vi "_PC_Daemon_Laser_Set_Status.vi"(5 "eng_mode_str":refnum<vi>, 7 "function":enum16{"none", "init", "set", "get"}(ring), 8 "error in (no error)":errorcluster, 10 "LaserSetting in":T1={"Energy"=50.0, "Freq"=100.0, "Emission"=FALSE, "TriggerSource"=enum."Internal", "Time Stamp"=timestamp(0 s since 1904-01-01)}, 11 "refnum cluster in":T2) -> (0 "error out":errorcluster, 2 "LaserSetting out":T1={"Energy"=50.0, "Freq"=100.0, "Emission"=FALSE, "TriggerSource"=enum."Internal", "Time Stamp"=timestamp(0 s since 1904-01-01)})   [LabVIEW 2018]
uses:
  RT/ControlLoop/Laser/Ctl/_ctl_LaserParam.ctl
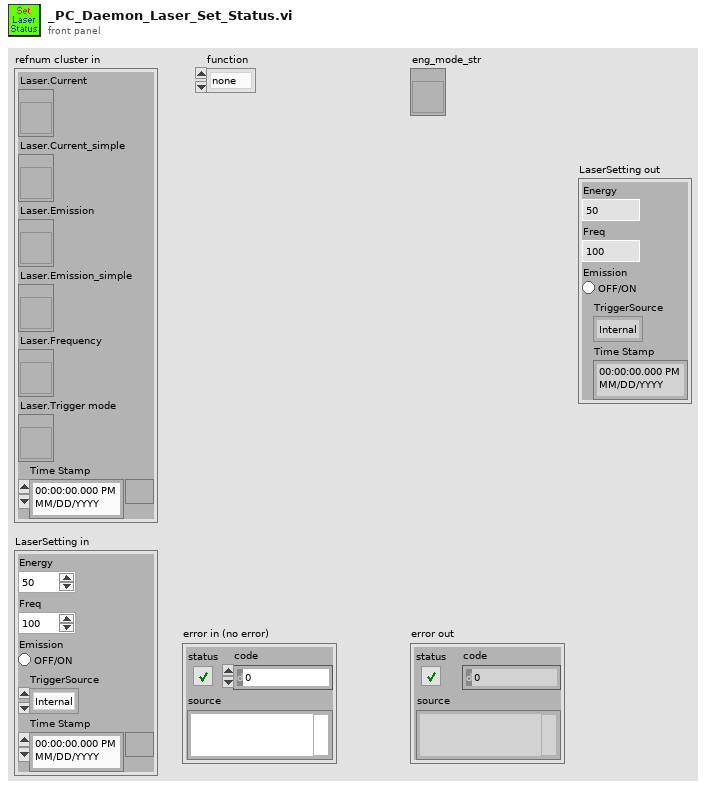
[diagram p1: front panel]
types:
  T1 = typedef "_ctl_LaserParam.ctl" = cluster{"Energy":dbl, "Freq":dbl, "Emission":bool, "TriggerSource":enum16{"Internal", "External"}, "Time Stamp":timestamp}
  T2 = cluster{"Laser.Current":refnum<vi>, "Laser.Current_simple":refnum<vi>, "Laser.Emission":refnum<vi>, "Laser.Emission_simple":refnum<vi>, "Laser.Frequency":refnum<vi>, "Laser.Trigger mode":refnum<vi>, "Time Stamp":timestamp}
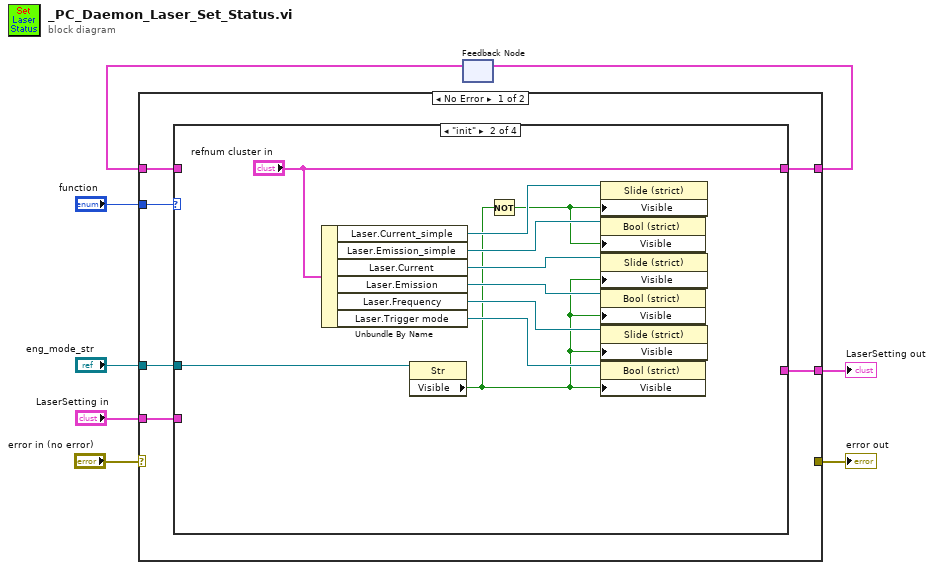
[diagram p0: block diagram]
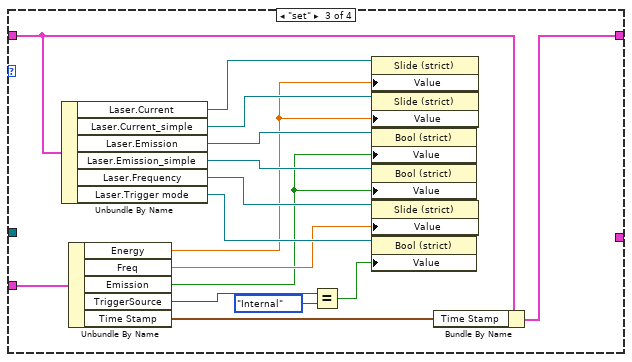
[diagram p3: hidden frame]
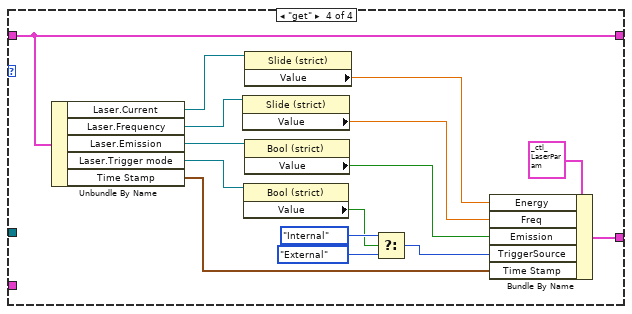
[diagram p4: hidden frame]
diagram:
  n1 = feedback #1() -> (w6:T2)  [unwired: 1 in]
  n2 = case shown="No Error" "error in (no error)" {
    selector: "error in (no error)" -> [_ w58]
    tunnel: "function" -> [w14 _]
    tunnel: [w13 w57] -> w7
    tunnel: w6 -> [w12 w57]
    tunnel: "eng_mode_str" -> [w11 _]
    tunnel: "LaserSetting in" -> [w10 _]
    tunnel: [_ w58] -> w2
    tunnel: [w9 _] -> w1
    frame No Error {
      n3 = case shown="\"init\"" w14 {
        tunnel: w12 -> [w15 _ w28 w56]
        tunnel: [w15 "refnum cluster in" w26 w56] -> w13
        tunnel: w11 -> [_ w25 _ _]
        tunnel: w10 -> [_ _ w35 _]
        tunnel: [_ _ _ w42] -> w9
        frame "none", Default {
        }
        frame "init" {
          n4 = Unbundle By Name("refnum cluster in") -> ("Laser.Current_simple"=w23:refnum<vi>, "Laser.Emission_simple"=w22:refnum<vi>, "Laser.Current"=w21:refnum<vi>, "Laser.Emission"=w20:refnum<vi>, "Laser.Frequency"=w19:refnum<vi>, "Laser.Trigger mode"=w18:refnum<vi>)
          n5 = property class="Str"(reference=w25) -> ("Visible"=w16:bool)  [unwired: 1 in, 2 out]
          n6 = Not(x=w16) -> (.not. x?=w17:bool)
          n7 = property class="Slide (strict)"(reference=w23, "Visible"=w17) -> ()  [unwired: 1 in, 2 out]
          n8 = property class="Bool (strict)"(reference=w22, "Visible"=w17) -> ()  [unwired: 1 in, 2 out]
          n9 = property class="Slide (strict)"(reference=w21, "Visible"=w16) -> ()  [unwired: 1 in, 2 out]
          n10 = property class="Bool (strict)"(reference=w20, "Visible"=w16) -> ()  [unwired: 1 in, 2 out]
          n11 = property class="Slide (strict)"(reference=w19, "Visible"=w16) -> ()  [unwired: 1 in, 2 out]
          n12 = property class="Bool (strict)"(reference=w18, "Visible"=w16) -> ()  [unwired: 1 in, 2 out]
        }
        frame "set" {
          n13 = Unbundle By Name(w28) -> ("Laser.Current"=w41:refnum<vi>, "Laser.Current_simple"=w40:refnum<vi>, "Laser.Emission"=w39:refnum<vi>, "Laser.Emission_simple"=w38:refnum<vi>, "Laser.Frequency"=w37:refnum<vi>, "Laser.Trigger mode"=w36:refnum<vi>)
          n14 = Unbundle By Name(w35) -> ("Energy"=w34:dbl, "Freq"=w33:dbl, "Emission"=w32:bool, "TriggerSource"=w30:enum16{"Internal", "External"}, "Time Stamp"=w27:timestamp)
          n15 = Equal?(x=w30, y=enum16{"Internal", "External"}."Internal" ("TriggerSource")) -> (x = y?=w29:bool)
          n16 = property class="Slide (strict)"(reference=w41, "Value"=w34) -> ()  [unwired: 1 in, 2 out]
          n17 = property class="Slide (strict)"(reference=w40, "Value"=w34) -> ()  [unwired: 1 in, 2 out]
          n18 = property class="Bool (strict)"(reference=w39, "Value"=w32) -> ()  [unwired: 1 in, 2 out]
          n19 = property class="Bool (strict)"(reference=w38, "Value"=w32) -> ()  [unwired: 1 in, 2 out]
          n20 = property class="Slide (strict)"(reference=w37, "Value"=w33) -> ()  [unwired: 1 in, 2 out]
          n21 = property class="Bool (strict)"(reference=w36, "Value"=w29) -> ()  [unwired: 1 in, 2 out]
          n22 = Bundle By Name(cluster=w28, "Time Stamp"=w27) -> (w26:T2)
        }
        frame "get" {
          n23 = Unbundle By Name(w56) -> ("Laser.Current"=w55:refnum<vi>, "Laser.Frequency"=w54:refnum<vi>, "Laser.Emission"=w53:refnum<vi>, "Laser.Trigger mode"=w52:refnum<vi>, "Time Stamp"=w46:timestamp)
          n24 = property class="Slide (strict)"(reference=w54) -> ("Value"=w45:dbl)  [unwired: 1 in, 2 out]
          n25 = property class="Bool (strict)"(reference=w52) -> ("Value"=w49:bool)  [unwired: 1 in, 2 out]
          n26 = property class="Slide (strict)"(reference=w55) -> ("Value"=w47:dbl)  [unwired: 1 in, 2 out]
          n27 = property class="Bool (strict)"(reference=w53) -> ("Value"=w44:bool)  [unwired: 1 in, 2 out]
          n28 = Select(t=enum16{"Internal", "External"}."Internal" ("TriggerSource"), s=w49, f=enum16{"Internal", "External"}."External" ("TriggerSource")) -> (s? t:f=w43:enum16{"Internal", "External"})
          n29 = Bundle By Name(cluster=T1 {"Energy"=50.0, "Freq"=100.0, "Emission"=FALSE, "TriggerSource"=enum."Internal", "Time Stamp"=timestamp(0 s since 1904-01-01)} ("LaserSetting"), "Energy"=w47, "Freq"=w45, "Emission"=w44, "TriggerSource"=w43, "Time Stamp"=w46) -> (w42:T1)
        }
      }
    }
    frame Error {
    }
  }
  "error out" <- w2
  "LaserSetting out" <- w1
  n30 = feedback-in #1(w7) -> ()
